vi "Collision Detection.vi"(9 "Keypress In":enum16{"Right", "Down", "Up", "Left"}(ring), 10 "Map In":u32[][](array[numeric]), 11 "Locations In":cluster{"Location Y":i32, "Location X":i32}[](array[cluster])=[{"Location Y"=12, "Location X"=8}, {"Location Y"=12, "Location X"=7}, {"Location Y"=12, "Location X"=6}, {"Location Y"=12, "Location X"=5}, {"Location Y"=12, "Location X"=4}]) -> (1 "Keypress Out":enum16{"Right", "Down", "Up", "Left"}(ring), 2 "Map Out":u32[][](array[numeric]), 3 "Locations Out":cluster{"Location Y":i32, "Location X":i32}[](array[cluster])=[{"Location Y"=12, "Location X"=8}, {"Location Y"=12, "Location X"=7}, {"Location Y"=12, "Location X"=6}, {"Location Y"=12, "Location X"=5}, {"Location Y"=12, "Location X"=4}], 4 "Collision?":bool, 5 "Game Over?":bool)   [LabVIEW 2014]
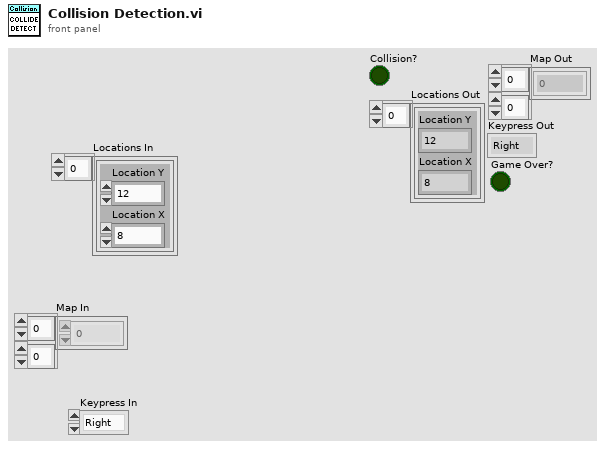
[diagram p1: front panel]
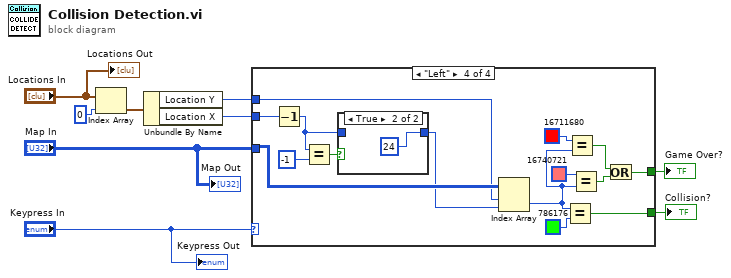
[diagram p0: block diagram]
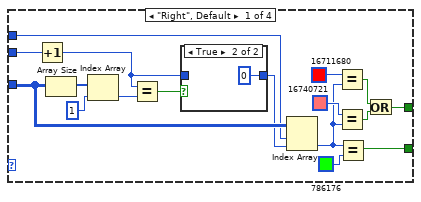
[diagram p2: hidden frame]
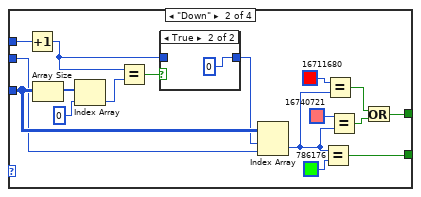
[diagram p4: hidden frame]
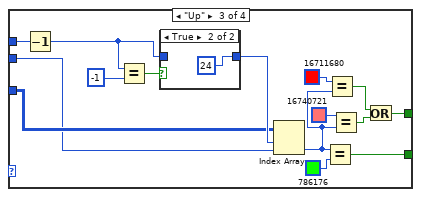
[diagram p6: hidden frame]
diagram:
  n1 = Index Array(array="Locations In", index=0) -> (element=w8:cluster{"Location Y":i32, "Location X":i32})
  n2 = Unbundle By Name(w8) -> ("Location Y"=w7:i32, "Location X"=w6:i32)
  n3 = case shown="\"Left\"" "Keypress In" {
    tunnel: w7 -> [w19 w45 w59 w77]
    tunnel: w6 -> [w20 w37 w53 w78]
    tunnel: "Map In" -> [w21 w40 w58 w79]
    tunnel: [w22 w31 w54 w65] -> w2
    tunnel: [w14 w30 w52 w66] -> w1
    frame "Right", Default {
      n4 = Increment(x=w20) -> (x+1=w17:i32)
      n5 = Array Size(array=w21) -> (size(s)=w26:i32[])
      n6 = Index Array(array=w26, index=1) -> (element=w24:i32)
      n7 = Equal?(x=w17, y=w24) -> (x = y?=w18:bool)
      n8 = case shown="True" w18 {
        tunnel: w17 -> [w27 _]
        tunnel: [w27 0] -> w16
        frame False {
        }
        frame True {
        }
      }
      n9 = Index Array(array=w21, index (row)=w19, index (col)=w16) -> (element=w11:u32)
      n10 = Equal?(x=u32 16711680, y=w11) -> (x = y?=w13:bool)
      n11 = Equal?(x=u32 16740721, y=w11) -> (x = y?=w12:bool)
      n12 = Equal?(x=w11, y=u32 786176) -> (x = y?=w22:bool)
      n13 = Or(x=w13, y=w12) -> (x .or. y?=w14:bool)
    }
    frame "Down" {
      n14 = Increment(x=w45) -> (x+1=w38:i32)
      n15 = Array Size(array=w40) -> (size(s)=w43:i32[])
      n16 = Index Array(array=w43, index=0) -> (element=w41:i32)
      n17 = Equal?(x=w38, y=w41) -> (x = y?=w44:bool)
      n18 = case shown="True" w44 {
        tunnel: w38 -> [w46 _]
        tunnel: [w46 0] -> w39
        frame False {
        }
        frame True {
        }
      }
      n19 = Index Array(array=w40, index (row)=w39, index (col)=w37) -> (element=w29:u32)
      n20 = Equal?(x=w29, y=u32 786176) -> (x = y?=w31:bool)
      n21 = Equal?(x=u32 16711680, y=w29) -> (x = y?=w34:bool)
      n22 = Equal?(x=u32 16740721, y=w29) -> (x = y?=w33:bool)
      n23 = Or(x=w34, y=w33) -> (x .or. y?=w30:bool)
    }
    frame "Up" {
      n24 = Decrement(x=w59) -> (x-1=w56:i32)
      n25 = Equal?(x=w56, y=-1 ("index")) -> (x = y?=w62:bool)
      n26 = case shown="True" w62 {
        tunnel: w56 -> [w63 _]
        tunnel: [w63 24] -> w61
        frame False {
        }
        frame True {
        }
      }
      n27 = Index Array(array=w58, index (row)=w61, index (col)=w53) -> (element=w49:u32)
      n28 = Equal?(x=w49, y=u32 786176) -> (x = y?=w54:bool)
      n29 = Equal?(x=u32 16711680, y=w49) -> (x = y?=w51:bool)
      n30 = Equal?(x=u32 16740721, y=w49) -> (x = y?=w50:bool)
      n31 = Or(x=w51, y=w50) -> (x .or. y?=w52:bool)
    }
    frame "Left" {
      n32 = Decrement(x=w78) -> (x-1=w74:i32)
      n33 = Equal?(x=w74, y=-1) -> (x = y?=w76:bool)
      n34 = case shown="True" w76 {
        tunnel: w74 -> [w80 _]
        tunnel: [w80 24] -> w73
        frame False {
        }
        frame True {
        }
      }
      n35 = Index Array(array=w79, index (row)=w77, index (col)=w73) -> (element=w67:u32)
      n36 = Equal?(x=w67, y=u32 786176) -> (x = y?=w65:bool)
      n37 = Equal?(x=u32 16711680, y=w67) -> (x = y?=w70:bool)
      n38 = Equal?(x=u32 16740721, y=w67) -> (x = y?=w69:bool)
      n39 = Or(x=w70, y=w69) -> (x .or. y?=w66:bool)
    }
  }
  "Collision?" <- w2
  "Game Over?" <- w1
  "Locations Out" <- "Locations In"
  "Map Out" <- "Map In"
  "Keypress Out" <- "Keypress In"
